vi "NIIE_Get Callers of Icon Editor Packed Library.vi"() -> (0 "CallersOfIconEditorPackedLibrary":path[](array[path]))   [LabVIEW 2021]
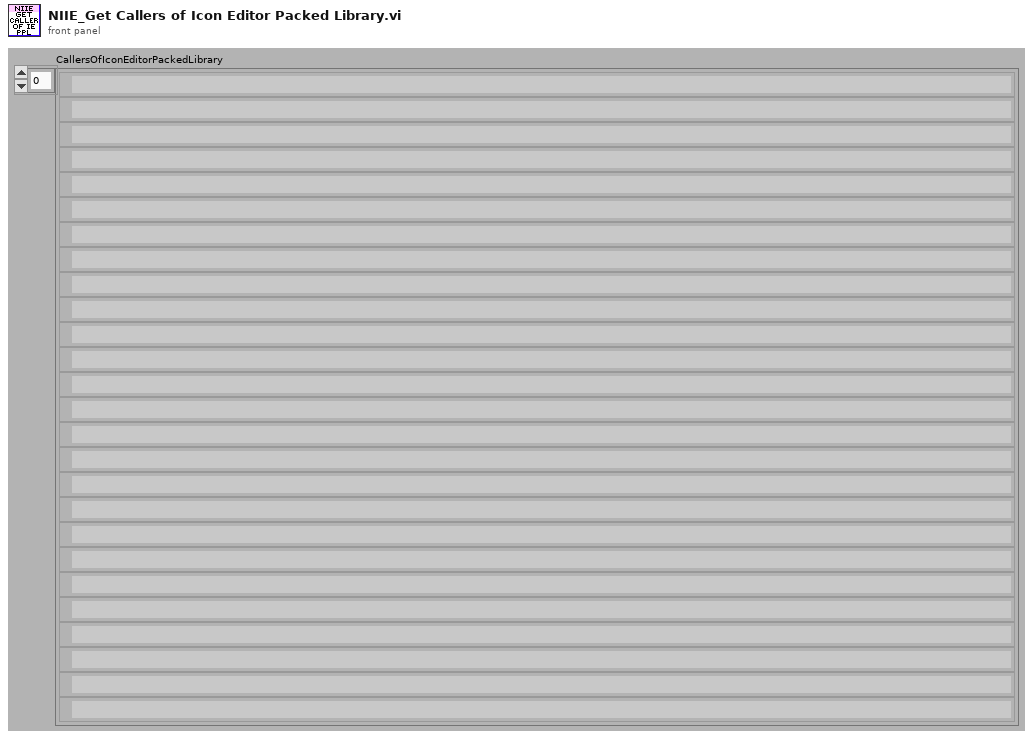
[diagram p1: front panel]
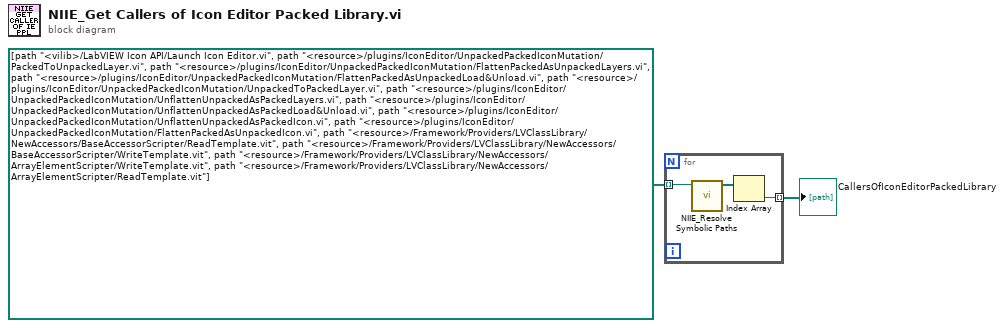
[diagram p0: block diagram]
diagram:
  n1 = for {
    tunnel: [w5] -> w2 mode=indexing
    tunnel: path[] [path "<vilib>/LabVIEW Icon API/Launch Icon Editor.vi", path "<resource>/plugins/IconEditor/UnpackedPackedIconMutation/PackedToUnpackedLayer.vi", path "<resource>/plugins/IconEditor/UnpackedPackedIconMutation/FlattenPackedAsUnpackedLayers.vi", path "<resource>/plugins/IconEditor/UnpackedPackedIconMutation/FlattenPackedAsUnpackedLoad&Unload.vi", path "<resource>/plugins/IconEditor/UnpackedPackedIconMutation/UnpackedToPackedLayer.vi", path "<resource>/plugins/IconEditor/UnpackedPackedIconMutation/UnflattenUnpackedAsPackedLayers.vi", path "<resource>/plugins/IconEditor/UnpackedPackedIconMutation/UnflattenUnpackedAsPackedLoad&Unload.vi", path "<resource>/plugins/IconEditor/UnpackedPackedIconMutation/UnflattenUnpackedAsPackedIcon.vi", path "<resource>/plugins/IconEditor/UnpackedPackedIconMutation/FlattenPackedAsUnpackedIcon.vi", path "<resource>/Framework/Providers/LVClassLibrary/NewAccessors/BaseAccessorScripter/ReadTemplate.vit", path "<resource>/Framework/Providers/LVClassLibrary/NewAccessors/BaseAccessorScripter/WriteTemplate.vit", path "<resource>/Framework/Providers/LVClassLibrary/NewAccessors/ArrayElementScripter/WriteTemplate.vit", path "<resource>/Framework/Providers/LVClassLibrary/NewAccessors/ArrayElementScripter/ReadTemplate.vit"] ("Array") -> [w4] mode=indexing
    n2 = call "NIIE_Resolve Symbolic Paths.vi"("symbolic path"=w4) -> ("resolved paths"=w3:path[])  [unwired: 10 in]
    n3 = Index Array(array=w3) -> (element=w5:path)  [unwired: 1 in]
  }
  "CallersOfIconEditorPackedLibrary" <- w2
